vi "borrowSyncComponentInterface.vi"(8 "error in (no error)":errorcluster, 11 "IBaseObject in":refnum<class "IBaseObject.lvclass">) -> (0 "error out":errorcluster, 2 "SyncComponent out":refnum<class "ISyncComponent.lvclass">, 3 "IBaseObject out":refnum<class "IBaseObject.lvclass">, 4 "err":u32)   [LabVIEW 2022 SP3, in "openDAQ.lvlib" / "IBaseObject.lvlib" / "IBaseObject.lvclass"]
uses:
  <instrlib>/openDAQ/Public/Classes/IBaseObject/IBaseObject.lvclass
  <instrlib>/openDAQ/Public/Classes/ISyncComponent/ISyncComponent.lvclass
  C:/Program Files (x86)/National Instruments/LabVIEW 2022/instr.lib/openDAQ/Public/Classes/IBaseObject/IBaseObject.lvclass
  <instrlib>/openDAQ/Public/Classes/IBaseObject/IBaseObject.lvclass/IBaseObject.ctl
  <instrlib>/openDAQ/Public/Classes/IBaseObject/Accessor/Read reference.vi
  <instrlib>/openDAQ/Public/Classes/IBaseObject/Accessor/Write reference.vi
  <instrlib>/openDAQ/Binaries/Windows/x86/copendaq32.dll
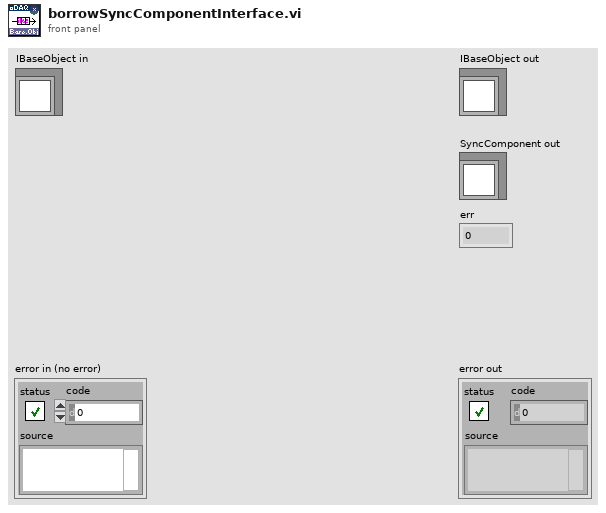
[diagram p1: front panel]
types:
  T1 = enum16{"big-endian, network order", "native, host order", "little-endian"}
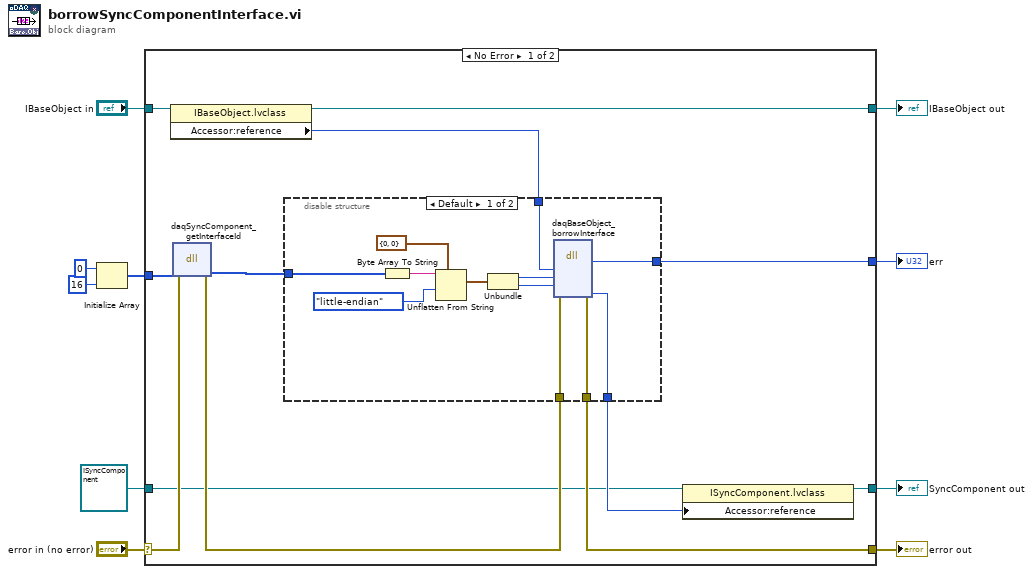
[diagram p0: block diagram]
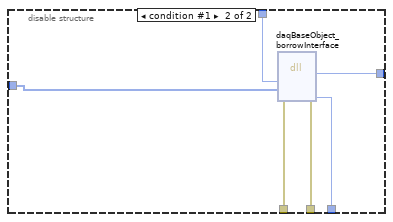
[diagram p2: hidden frame]
diagram:
  n1 = Initialize Array(u8 0, 16 ("dimension size")) -> (w2:u8[])
  n2 = case shown="No Error" "error in (no error)" {
    selector: "error in (no error)" -> [w19 w43]
    tunnel: [w21 w43] -> w9
    tunnel: [w12 w42] -> w7
    tunnel: "IBaseObject in" -> [w22 w42]
    tunnel: refnum<class "ISyncComponent.lvclass"> refnum ("openDAQ.lvlib:IBaseObject.lvlib:IPropertyObject.lvlib:IComponent.lvlib:ISyncComponent.lvlib:ISyncComponent.lvclass") -> [w13 w41]
    tunnel: w2 -> [w17 _]
    tunnel: [w15 w41] -> w5
    tunnel: [w11 _] -> w1
    frame No Error {
      n3 = property class="IBaseObject.lvclass"(reference=w22) -> (reference out=w12:refnum<class "IBaseObject.lvclass">, "Accessor:reference"=w20:i64)  [unwired: 1 in, 1 out]
      n4 = dll-call lib="C:/Program Files (x86)/National Instruments/LabVIEW 2022/instr.lib/openDAQ/Binaries/Windows/x86/copendaq*.*" fn="daqSyncComponent_getInterfaceId"(error in=w19, "id"=w17) -> (error out=w18:errorcluster, "id"=w14:u8[])  [unwired: 3 in, 1 out]
      n5 = disable-structure shown="Default" {
        disable-tunnel: [w34 w39] -> w21
        disable-tunnel: w20 -> [w24 w35]
        disable-tunnel: w18 -> [w33 w40]
        disable-tunnel: [w32 w38] -> w16
        disable-tunnel: w14 -> [w28 w37]
        disable-tunnel: [w23 w36] -> w11
        frame condition #0 (active) {
          n6 = Byte Array To String(unsigned byte array=w28) -> (string=w31:string)
          n7 = Unflatten From String(type=cluster{u64, u64} {0, 0}, binary string=w31, byte order (0:big-endian, network order)=T1."little-endian") -> (value=w29:cluster{u64, u64})  [unwired: 2 in, 2 out]
          n8 = Unbundle(w29) -> (w27:u64, w26:u64)
          n9 = dll-call lib="C:/Program Files (x86)/National Instruments/LabVIEW 2022/instr.lib/openDAQ/Binaries/Windows/x86/copendaq*.*" fn="daqBaseObject_borrowInterface"(error in=w33, "self"=w24, "intfId1"=w27, "intfId2"=w26) -> (error out=w34:errorcluster, "return type"=w23:u32, "interfacePtr"=w32:i64)  [unwired: 6 in, 1 out]
        }
        frame condition #1 {
          n10 = dll-call lib="C:/Program Files (x86)/National Instruments/LabVIEW 2022/instr.lib/openDAQ/Binaries/Windows/x86/copendaq*.*" fn="daqBaseObject_borrowInterface"(error in=w40, "self"=w35, "intfId"=w37) -> (error out=w39:errorcluster, "return type"=w36:u32, "interfacePtr"=w38:i64)  [unwired: 5 in, 1 out]
        }
      }
      n11 = property class="ISyncComponent.lvclass"(reference=w13, "Accessor:reference"=w16) -> (reference out=w15:refnum<class "ISyncComponent.lvclass">)  [unwired: 1 in, 1 out]
    }
    frame Error {
    }
  }
  "error out" <- w9
  "IBaseObject out" <- w7
  "SyncComponent out" <- w5
  "err" <- w1
